vi "Reset Limits Multicolumn Listbox.vi"(8 "error in (no error)":errorcluster, 11 "Cluster in":T1) -> (0 "error out":errorcluster)   [LabVIEW 2019, in "ZenGage v3.0 UI.lvclass"]
uses:
  ZenGage v3.0 UI.lvclass
  <vilib>/Utility/miscctls.llb/LVRowAndColumnTypeDef.ctl
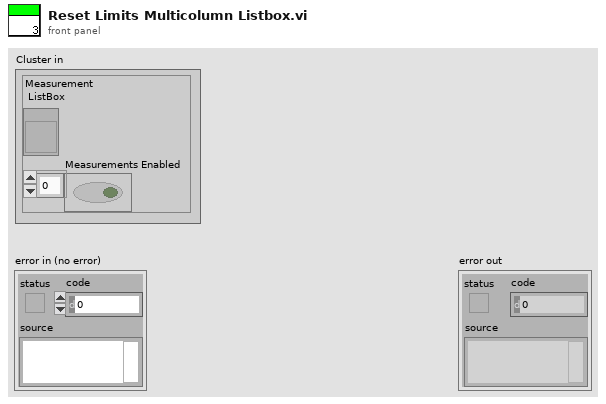
[diagram p1: front panel]
types:
  T1 = cluster{"Measurement\n ListBox":refnum<vi>, "Measurements Enabled":bool[]}
  T2 = typedef "LVRowAndColumnTypeDef.ctl" = cluster{"Row":i32, "Column":i32}
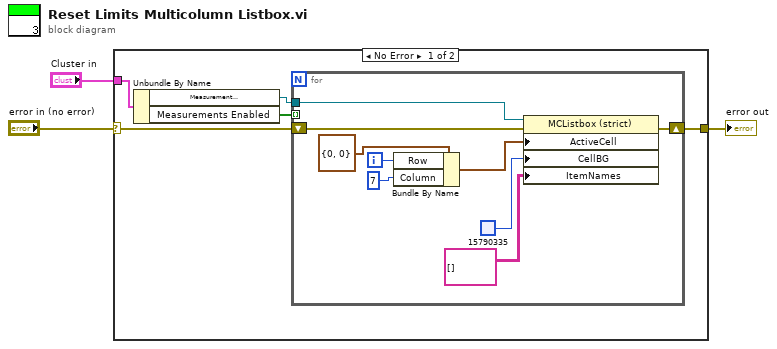
[diagram p0: block diagram]
diagram:
  n1 = case shown="No Error" "error in (no error)" {
    selector: "error in (no error)" -> [w5 w18]
    tunnel: [w4 w18] -> w2
    tunnel: "Cluster in" -> [w8 _]
    frame No Error {
      n2 = Unbundle By Name(w8) -> ("Measurement\n ListBox"=w6:refnum<vi>, "Measurements Enabled"=w7:bool[])
      n3 = for {
        tunnel: w7 -> [_] mode=indexing
        tunnel: w6 -> [w17]
        shift-right: [w12] -> w4
        shift-left: w5 -> [w11]
        i -> [w14]
        n4 = Bundle By Name(cluster=T2 {"Row"=0, "Column"=0} ("Active Cell:Active Cell"), "Row"=w14, "Column"=7) -> (w15:T2)
        n5 = property class="MCListbox (strict)"(reference=w17, error in=w11, "ActiveCell"=w15, "CellBG"=u32 15790335, "ItemNames"=string[][] [] ("Item Names")) -> (error out=w12:errorcluster)  [unwired: 1 out]
      }
    }
    frame Error {
    }
  }
  "error out" <- w2
